vi "SimpleProgram.vi"() -> ()   [LabVIEW 2018, in "JULABO DeviceDriver.lvlib"]
doc: "Basic example how to read temperatures and adjust setpoint"
uses:
  JULABO DeviceDriver.lvlib
panel:
  in  "StartStop":bool
  out "Numerisch":i32
  out "device error out":errorcluster
  out "Diagram":T1(graph)
  in  "Read cycle (ms)":u32=1000
  in  "ID Query? (T: Yes)":bool=TRUE
  in  "RS485-Address (128: RS232)":u32=128
  in  "VISA resource name":refnum<visa-resource-name>="COM3"
  in  "Serial Configuration":T2={"Baud Rate"=4800, "Parity"=2, "Data Bits"=7, "Stop Bits"=10, "Flow Control"=2} {"Flow Control" items=["None", "XON/XOFF", "RTS/CTS", "XON/XOFF & RTS/CTS", "DTR/DSR", "XON/XOFF & DTR/DSR"]; "Stop Bits" items=["1.0"=10, "1.5"=15, "2.0"=20]; "Data Bits" items=["7"=7, "8"=8]; "Parity" items=["None", "Odd", "Even", "Mark", "Space"]; "Baud Rate" items=["300"=300, "600"=600, "1200"=1200, "2400"=2400, "4800"=4800, "9600"=9600, "19200"=19200]}
  in  "Reset / Default (T: Both)":bool=TRUE
  in  "Stop":bool
  out "Power":i8(slide) scale=-100.0..100.0
  out "InternalTemp":dbl format="%.2f"
  in  "Setpoint":dbl format="%.2f"
  # "1. Select the COM-Port and adjust the serial\nconfiguration for your instrument\n2. Adjust the Read cycle\n3. Start the VI by pressing the \"Start\" -Button\n( Arrow button on the top-left corner)\n4. To stop the execution press the \"Stop\" button"
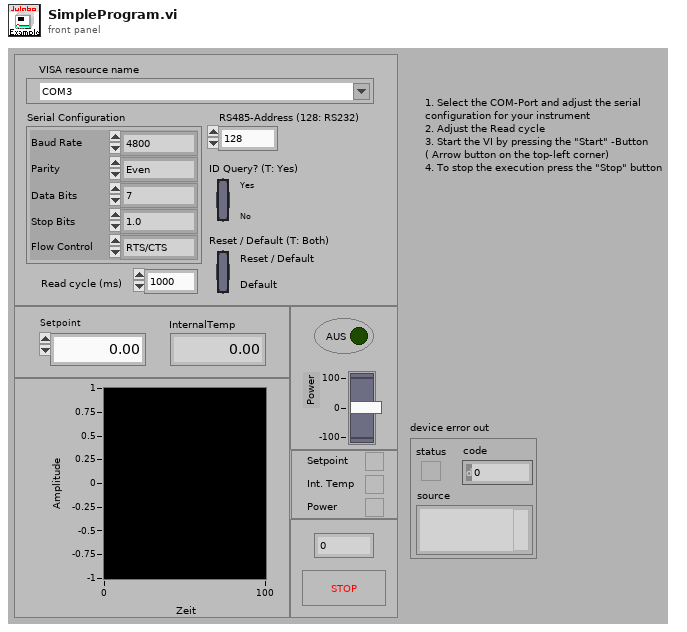
[diagram p1: front panel]
types:
  T1 = cluster{"Setpoint":dbl, "InternalTemp (out)":dbl, "Capacity (out)":i8}
  T2 = cluster{"Baud Rate":u32, "Parity":u16, "Data Bits":u16, "Stop Bits":u16, "Flow Control":u16}
  T3 = cluster{"Setpoint (out)":dbl, "InternalTemp (out)":dbl, "Capacity (out)":i8}
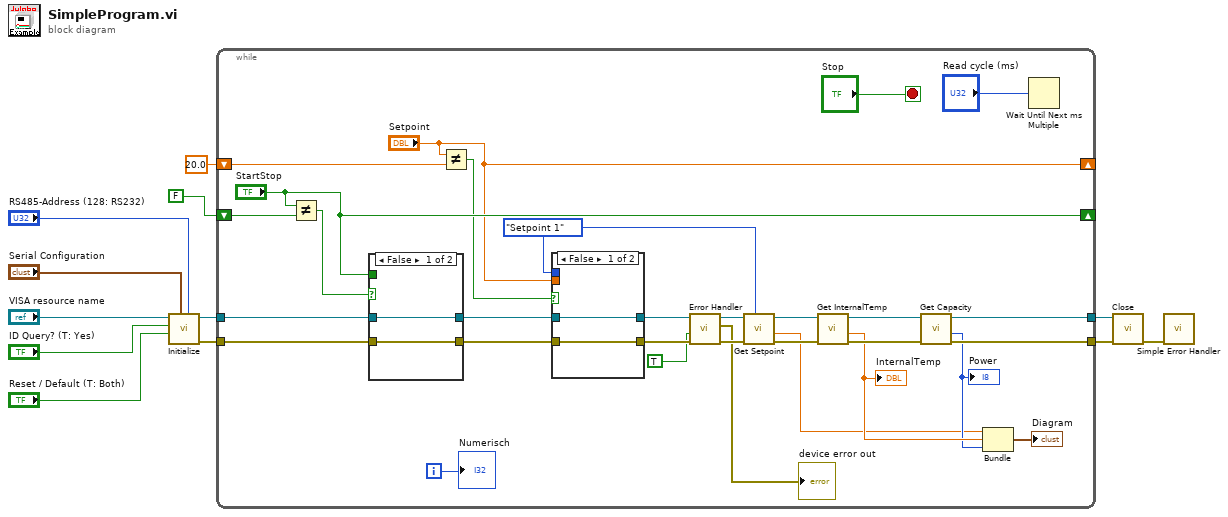
[diagram p0: block diagram]
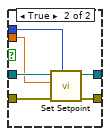
[diagram p2: hidden frame]
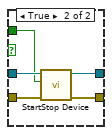
[diagram p3: hidden frame]
diagram:
  n1 = call "Initialize.vi"("RS485-Address (128: RS232)"="RS485-Address (128: RS232)", "Serial Configuration"="Serial Configuration", "Reset / Default (T: Both)"="Reset / Default (T: Both)", "ID Query? (T: Yes)"="ID Query? (T: Yes)", "VISA resource name"="VISA resource name") -> ("error out"=w9:errorcluster, "VISA resource name out"=w12:refnum<visa-resource-name>)  [unwired: 5 in]
  n2 = while {
    tunnel: w12 -> [w20]
    tunnel: [w41] -> w11
    tunnel: [w40] -> w10
    tunnel: w9 -> [w19]
    shift-right: ["StartStop"] -> _
    shift-left: FALSE ("StartStop") -> [w18]
    shift-right: ["Setpoint"] -> _
    shift-left: 20.0 ("Setpoint") -> [w15]
    i -> [w23]
    stop <- "Stop" stop-if-true
    w27 = enum16{"Setpoint 1", "Setpoint 2", "Setpoint 3"}."Setpoint 1" ("Setpoint")
    n3 = Not Equal?(x="StartStop", y=w18) -> (x != y?=w17:bool)
    n4 = case shown="False" w17 {
      tunnel: [w52 w57] -> w22
      tunnel: [w51 w56] -> w21
      tunnel: w20 -> [w52 w55]
      tunnel: w19 -> [w51 w54]
      tunnel: "StartStop" -> [_ w53]
      frame False {
      }
      frame True {
        n5 = call "StartStop Device.vi"("error in (no error)"=w54, "Start/Stop (f:Stop)"=w53, "VISA resource name"=w55) -> ("error out"=w56:errorcluster, "VISA resource name out"=w57:refnum<visa-resource-name>)  [unwired: 7 in]
      }
    }
    n6 = Not Equal?(x="Setpoint", y=w15) -> (x != y?=w14:bool)
    n7 = case shown="False" w14 {
      tunnel: [w43 w50] -> w33
      tunnel: [w44 w49] -> w32
      tunnel: w27 -> [_ w45]
      tunnel: w22 -> [w44 w48]
      tunnel: w21 -> [w43 w47]
      tunnel: "Setpoint" -> [_ w46]
      frame False {
      }
      frame True {
        n8 = call "Set Setpoint.vi"("Setpointindex (Setpoint1: Default)"=w45, "error in (no error)"=w47, "newSetpoint (20.00°C)"=w46, "VISA resource name"=w48) -> ("error out"=w50:errorcluster, "VISA resource name out"=w49:refnum<visa-resource-name>)  [unwired: 6 in]
      }
    }
    n9 = call "Error Handler.vi"("error in (no error)"=w33, "ClearCommandError (false)"=TRUE, "VISA resource name"=w32) -> ("error out"=w25:errorcluster, "device error out"=→"device error out":errorcluster, "VISA resource name out"=w31:refnum<visa-resource-name>)  [unwired: 5 in, 1 out]
    n10 = call "Get Setpoint.vi"("Setpointindex"=w27, "error in (no error)"=w25, "VISA resource name"=w31) -> ("error out"=w29:errorcluster, "Setpoint (out)"=w28:dbl, "VISA resource name out"=w30:refnum<visa-resource-name>)  [unwired: 6 in]
    n11 = call "Get InternalTemp.vi"("error in (no error)"=w29, "VISA resource name"=w30) -> ("error out"=w39:errorcluster, "InternalTemp (out)"=w37:dbl, "VISA resource name out"=w42:refnum<visa-resource-name>)  [unwired: 7 in]
    "InternalTemp" <- w37
    n12 = call "Get Capacity.vi"("error in (no error)"=w39, "VISA resource name"=w42) -> ("error out"=w40:errorcluster, "Capacity (out)"=w36:i8, "VISA resource name out"=w41:refnum<visa-resource-name>)  [unwired: 7 in]
    "Power" <- w36
    n13 = Bundle("Setpoint (out)"=w28, "InternalTemp (out)"=w37, "Capacity (out)"=w36) -> (→"Diagram":T3)  [unwired: 1 in]
    n14 = Wait Until Next ms Multiple(millisecond multiple="Read cycle (ms)") -> ()  [unwired: 1 out]
    "Numerisch" <- w23
  }
  n15 = call "Close.vi"("error in (no error)"=w10, "VISA resource name"=w11) -> ("error out"=w6:errorcluster)  [unwired: 9 in]
  n16 = call <vilib>:"Simple Error Handler.vi"("error in (no error)"=w6) -> ()  [unwired: 4 in, 5 out]
